vi "JoystickRumblePatternControl.vi"(2 "RumblePeriod(ms)":sgl=1000.0, 3 "RumbleIntensity":sgl=1.0, 4 "RumbleMode":T1) -> (0 "RightRumble":sgl, 1 "LeftRumble":sgl)   [LabVIEW 2019, in "ArgosLib.lvlib"]
uses:
  ArgosLib.lvlib
  TypeDefs/JSRumbleMode.ctl
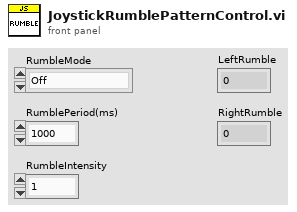
[diagram p1: front panel]
types:
  T1 = typedef "ArgosLib.lvlib/JSRumbleMode.ctl" = enum16{"Off", "On", "Pulse", "Alternate", "SmoothPulse", "SmoothAlternate"}
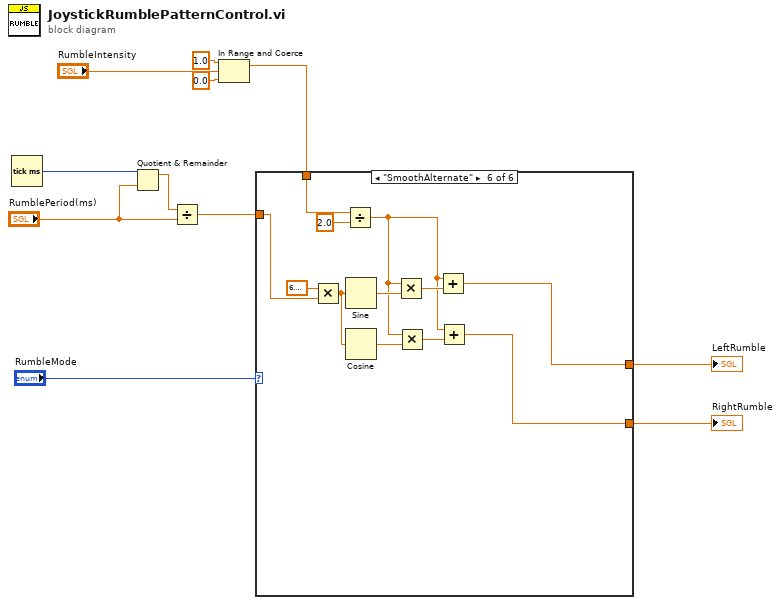
[diagram p0: block diagram]
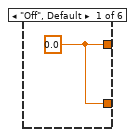
[diagram p2: hidden frame]
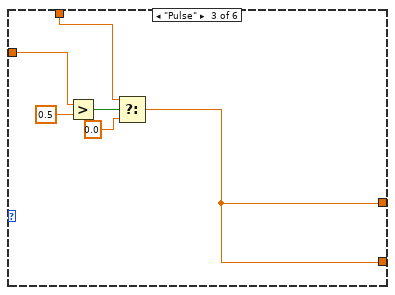
[diagram p4: hidden frame]
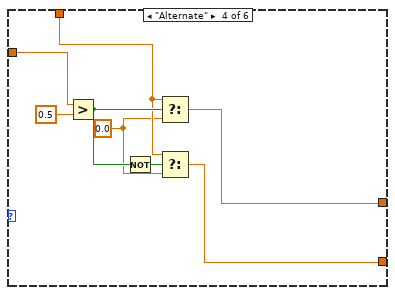
[diagram p5: hidden frame]
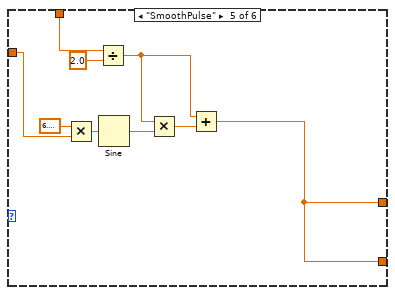
[diagram p6: hidden frame]
diagram:
  n1 = Tick Count (ms)() -> (millisecond timer value=w11:u32)
  n2 = Quotient & Remainder(x=w11, y="RumblePeriod(ms)") -> (x-y*floor(x/y)=w10:sgl)  [unwired: 1 out]
  n3 = Divide(x=w10, y="RumblePeriod(ms)") -> (x/y=w1:sgl)
  n4 = In Range and Coerce(upper limit=sgl 1.0, x="RumbleIntensity", lower limit=sgl 0.0) -> (coerced(x)=w4:sgl)  [unwired: 1 out]
  n5 = case shown="\"SmoothAlternate\"" "RumbleMode" {
    tunnel: [w12 w13 w14 w25 w28 w42] -> w7
    tunnel: [w12 w13 w14 w20 w28 w37] -> w6
    tunnel: w4 -> [_ w13 w16 w22 w33 w46]
    tunnel: w1 -> [_ _ w19 w27 w35 w48]
    frame "Off", Default {
      w12 = 0.0 ("LeftRumble")
    }
    frame "On" {
    }
    frame "Pulse" {
      n6 = Greater?(x=w19, y=0.5) -> (0:w17:bool)
      n7 = Select(t=w16, s=w17, f=0.0) -> (s? t:f=w14:dbl)
    }
    frame "Alternate" {
      w21 = 0.0 ("f")
      n8 = Greater?(x=w27, y=0.5) -> (0:w23:bool)
      n9 = Not(x=w23) -> (.not. x?=w24:bool)
      n10 = Select(t=w22, s=w23, f=w21) -> (s? t:f=w25:dbl)
      n11 = Select(t=w22, s=w24, f=w21) -> (s? t:f=w20:dbl)
    }
    frame "SmoothPulse" {
      n12 = Multiply(x=6.283185307179586, y=w35) -> (x*y=w36:dbl)
      n13 = Divide(x=w33, y=2.0) -> (x/y=w29:dbl)
      n14 = Sine(x=w36) -> (sin(x)=w31:dbl)
      n15 = Multiply(x=w29, y=w31) -> (x*y=w30:dbl)
      n16 = Add(x=w29, y=w30) -> (x+y=w28:dbl)
    }
    frame "SmoothAlternate" {
      n17 = Multiply(x=sgl 6.2831855, y=w48) -> (x*y=w41:sgl)
      n18 = Divide(x=w46, y=sgl 2.0) -> (x/y=w38:sgl)
      n19 = Sine(x=w41) -> (sin(x)=w44:sgl)
      n20 = Cosine(x=w41) -> (cos(x)=w39:sgl)
      n21 = Multiply(x=w38, y=w44) -> (x*y=w43:sgl)
      n22 = Multiply(x=w38, y=w39) -> (x*y=w40:sgl)
      n23 = Add(x=w38, y=w43) -> (x+y=w42:sgl)
      n24 = Add(x=w38, y=w40) -> (x+y=w37:sgl)
    }
  }
  "LeftRumble" <- w7
  "RightRumble" <- w6
